vi "NotifyIcon - Set ContextMenu.vi"(8 "error in":errorcluster, 10 "Context Menu":string[][](array[string]), 11 "NotifyIcon reference in":refnum<k24>) -> (0 "error out":errorcluster, 3 "NotifyIcon reference out":refnum<k24>)   [LabVIEW 2020]
doc: "Sets a pop-up menu that will be shown when the Icon is right-clicked.\n\nIn order to capture events from this menu, use NotifyIcon - Register LabVIEW User Events.vi or use the .NET API."
uses:
  System.Windows.Forms
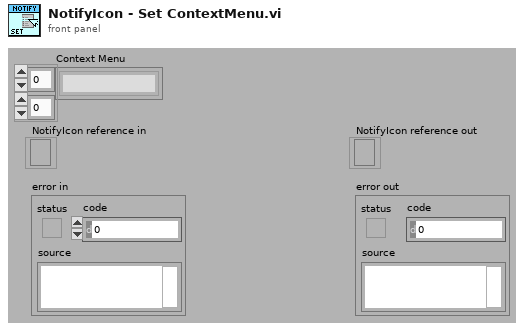
[diagram p1: front panel]
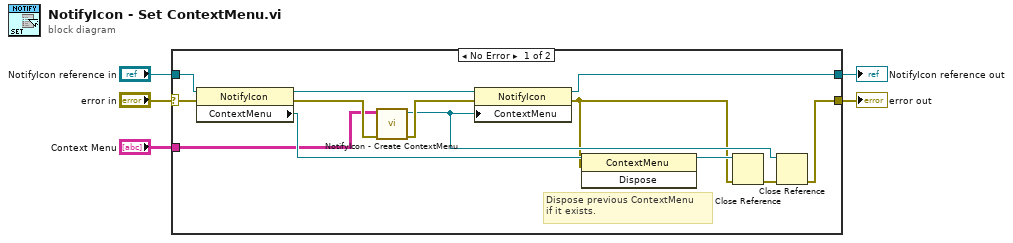
[diagram p0: block diagram]
diagram:
  n1 = case shown="No Error" "error in" {
    selector: "error in" -> [w11 w19]
    tunnel: [w18 w20] -> w5
    tunnel: "NotifyIcon reference in" -> [w17 w20]
    tunnel: [w6 w19] -> w3
    tunnel: "Context Menu" -> [w12 _]
    frame No Error {
      # "Dispose previous ContextMenu\nif it exists."
      n2 = property class="NotifyIcon"(reference=w17, error in=w11) -> (reference out=w16:refnum<k24>, error out=w14:errorcluster, "ContextMenu"=w15:refnum<k24>)
      n3 = call "NotifyIcon - Create ContextMenu.vi"("error in"=w14, "Menus"=w12) -> ("error out"=w13:errorcluster, "ContextMenu reference"=w9:refnum<k24>)  [unwired: 8 in]
      n4 = property class="NotifyIcon"(reference=w16, error in=w13, "ContextMenu"=w9) -> (reference out=w18:refnum<k24>, error out=w7:errorcluster)
      n5 = invoke class="ContextMenu" method="Dispose"(reference=w15, error in=w7) -> (reference out=w10:refnum<k24>)  [unwired: 1 in, 2 out]
      n6 = Close Reference(reference=w10, error in (no error)=w7) -> (error out=w8:errorcluster)
      n7 = Close Reference(reference=w9, error in (no error)=w8) -> (error out=w6:errorcluster)
    }
    frame Error {
    }
  }
  "NotifyIcon reference out" <- w5
  "error out" <- w3
